vi "Init Spark Max With CVS File.vi"(3 "error in":errorcluster, 4 "Motor ID":string="Winch", 5 "Robot ID":string="981") -> (0 "error out":errorcluster, 2 "CAN Talon SRX Ref":T1={"DeviceStatus"={"status"=FALSE, "code"=0, "source"=""}, "Type"=enum."PWM", "PWM"={"PWM Channel"=enum."PWM 1", "DeadBand"={"Name"="", "maxPositivePwm"=0, "minPositivePwm"=0, "centerPwm"=0, "maxNegativePwm"=0, "minNegativePwm"=0, "angularRange"=0}}, "CAN"={"Device Number"=0, "SetOutput VI Ref"=variant(enum8{"Percent VBus", "Current", "Speed", "Position", "Voltage"} enum."Percent VBus"), "GetOutput VI Ref"=variant(refnum<k1> refnum), "Enable VI Ref"=variant(dbl 12.0), "Disable VI Ref"=variant(enum8{"Percent VBus", "Speed", "Position", "Slave", "Unchanged / Invalid", "Voltage Compensation", "Current", "Motion Profile"} enum."Percent VBus"), "Data"=variant}, "Invert"=FALSE, "DIO PWM"={"PWM \"Enable\" Channel"=enum."Invalid", "DIOChannel"=enum."Invalid", "PWM Rate"=0.0}})   [LabVIEW 2020]
uses:
  <vilib>/Rock Robotics/WPI/MotorControl/WPI_MotorControlDeviceRef.ctl
  <vilib>/Rock Robotics/WPI/MotorControl/WPI_MotorControlType.ctl
  <vilib>/Rock Robotics/SystemInterfaces/DIO/FPGA_DIOPWMChannel.ctl
  <vilib>/Rock Robotics/WPI/PWM/WPI_PWMDeadband.ctl
  <vilib>/Rock Robotics/SystemInterfaces/DIO/FPGA_DIOChannel.ctl
  2022 Robot Global Data.vi
  2023 Robot Global Data.vi
panel:
  out "Motor ID 2":string="Winch"
  out "CVS Provided CAN Bus ID":u8
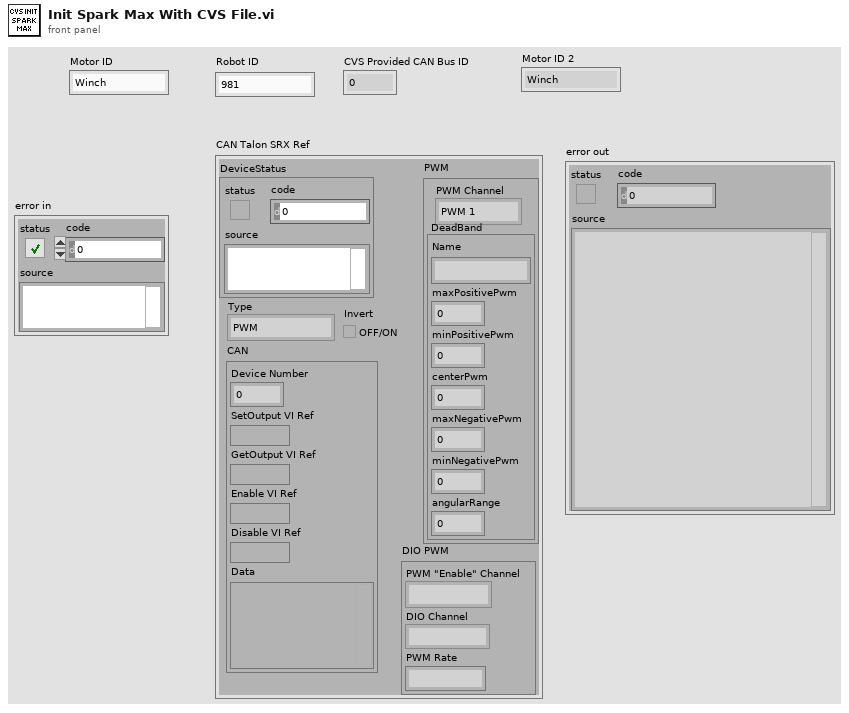
[diagram p1: front panel]
types:
  T1 = typedef "WPI_MotorControlDeviceRef.ctl" = cluster{"DeviceStatus":errorcluster, "Type":T2, "PWM":cluster{"PWM Channel":T3, "DeadBand":T4}, "CAN":cluster{"Device Number":u8, "SetOutput VI Ref":variant, "GetOutput VI Ref":variant, "Enable VI Ref":variant, "Disable VI Ref":variant, "Data":variant}, "Invert":bool, "DIO PWM":cluster{"PWM \"Enable\" Channel":T3, "DIOChannel":T5, "PWM Rate":dbl}}
  T2 = typedef "WPI_MotorControlType.ctl" = enum16{"PWM", "CAN", "DIO PWM"}
  T3 = typedef "FPGA_DIOPWMChannel.ctl" = enum8{"PWM 0", "PWM 1", "PWM 2", "PWM 3", "PWM 4", "PWM 5", "PWM 6", "PWM 7", "PWM 8", "PWM 9", "PWM MXP 0", "PWM MXP 1", "PWM MXP 2", "PWM MXP 3", "PWM MXP 4", "PWM MXP 5", "PWM MXP 6", "PWM MXP 7", "PWM MXP 8", "PWM MXP 9", "Invalid"}
  T4 = typedef "WPI_PWMDeadband.ctl" = cluster{"Name":string, "maxPositivePwm":i32, "minPositivePwm":i32, "centerPwm":i32, "maxNegativePwm":i32, "minNegativePwm":i32, "angularRange":u16}
  T5 = typedef "FPGA_DIOChannel.ctl" = enum8{"DIO 0", "DIO 1", "DIO 2", "DIO 3", "DIO 4", "DIO 5", "DIO 6", "DIO 7", "DIO 8", "DIO 9", "DIO MXP 0", "DIO MXP 1", "DIO MXP 2", "DIO MXP 3", "DIO MXP 4", "DIO MXP 5", "DIO MXP 6", "DIO MXP 7", "DIO MXP 8", "DIO MXP 9", "DIO MXP 10", "DIO MXP 11", "DIO MXP 12", "DIO MXP 13", "DIO MXP 14", "DIO MXP 15", "SPI Port CS1", "SPI Port CS2", "SPI Port CS3", "SPI Port MISO", "SPI Port MOSI", "Invalid"}
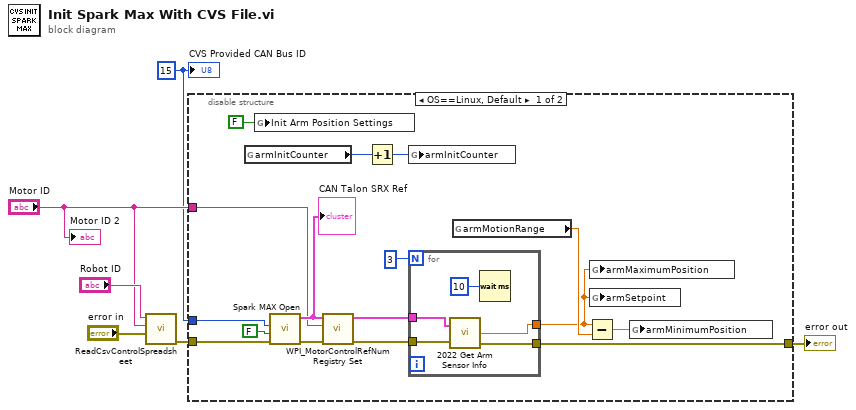
[diagram p0: block diagram]
diagram:
  w1 = u8 15 ("CVS Provided CAN Bus ID")
  n1 = call "ReadCsvControlSpreadsheet.vi"("error in"="error in", "Motor ID"="Motor ID", "Robot ID"="Robot ID") -> ("error out"=w4:errorcluster)  [unwired: 8 out]
  n2 = disable-structure shown="OS==Linux, Default" {
    disable-tunnel: "Motor ID" -> [w18 _]
    disable-tunnel: w4 -> [w22 w28]
    disable-tunnel: [w10 w28] -> w3
    disable-tunnel: w1 -> [w21 _]
    frame condition #0 (active) {
      n3 = global read "2022 Robot Global Data.vi" "armInitCounter"() -> (w7:i32)
      n4 = global write "2022 Robot Global Data.vi" "Init Arm Position Settings"(FALSE ("First Time")) -> ()
      n5 = call <vilib>:"Spark MAX Open.vi"("error in (no error)"=w22, "Invert"=FALSE, "Device Number"=w21) -> ("error out"=w20:errorcluster, "MotorControlDeviceRef"=w19:T1)  [unwired: 7 in]
      "CAN Talon SRX Ref" <- w19
      n6 = call <vilib>:"WPI_MotorControlRefNum Registry Set.vi"("error in (no error)"=w20, "refnum name"=w18, "MotorControlDevRef"=w19) -> ("error out"=w12:errorcluster, "MotorControlDevRef"=w13:T1)  [unwired: 7 in]
      n7 = Increment(x=w7) -> (x+1=w8:i32)
      n8 = global write "2022 Robot Global Data.vi" "armInitCounter"(w8) -> ()
      n9 = for {
        N: 3 -> [_]
        tunnel: w13 -> [w26]
        tunnel: w12 -> [w25]
        tunnel: [w24] -> w11
        tunnel: [w23] -> w10
        n10 = call "2022 Get Arm Sensor Info.vi"("MotorControlDevRefIn"=w26, "error in (no error)"=w25) -> ("armSensorPosition"=w24:dbl, "error out"=w23:errorcluster)  [unwired: 1 out]
        n11 = Wait (ms)(milliseconds to wait=u32 10) -> ()  [unwired: 1 out]
      }
      n12 = global read "2023 Robot Global Data.vi" "armMotionRange"() -> (w16:dbl)
      n13 = Subtract(x=w11, y=w16) -> (x-y=w15:dbl)
      n14 = global write "2023 Robot Global Data.vi" "armMaximumPosition"(w11) -> ()
      n15 = global write "2023 Robot Global Data.vi" "armSetpoint"(w11) -> ()
      n16 = global write "2023 Robot Global Data.vi" "armMinimumPosition"(w15) -> ()
    }
    frame condition #1 {
    }
  }
  "error out" <- w3
  "CVS Provided CAN Bus ID" <- w1
  "Motor ID 2" <- "Motor ID"
